vi "Excel - Close Docuement Tests.vi"(8 "error in (no error)":errorcluster) -> (0 "error out":errorcluster)   [LabVIEW 2017]
uses:
  src/LabVIEW NPOI/MS-Excel/MS-Excel.lvclass
  src/LabVIEW NPOI/Document/Document.lvclass
  <vilib>/addons/_JKI Toolkits/Caraya/classes/Test/Test.lvclass
  <vilib>/addons/_JKI Toolkits/Caraya/classes/Assert/Assert.lvclass
  <vilib>/addons/_JKI Toolkits/Caraya/classes/Assert/Assert Not Error.vi
  <vilib>/addons/_JKI Toolkits/Caraya/classes/Assert/Assert True.vi
  D:/Benjamin/Documents/Perso/Code/WC/LabVIEW_NPOI/src/LabVIEW NPOI/Document/Document.lvclass
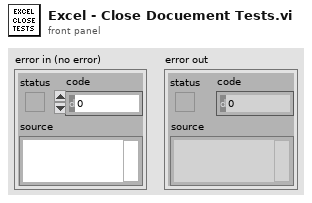
[diagram p1: front panel]
types:
  T1 = enum16{"open", "replace", "create", "open or create", "replace or create", "replace or create with confirmation"}
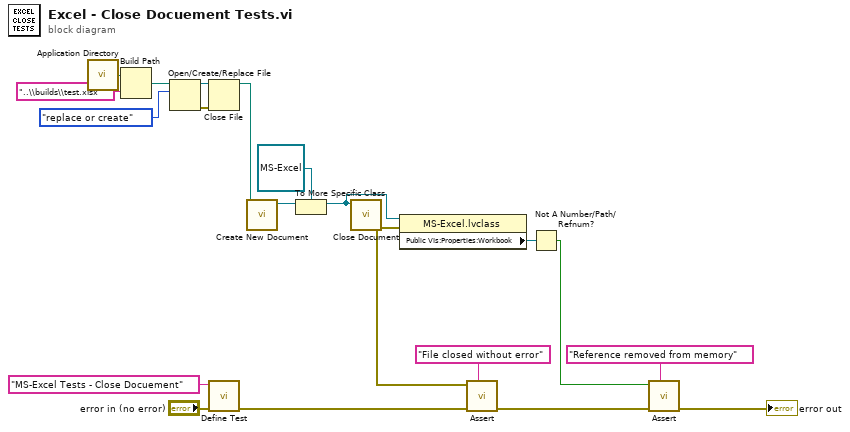
[diagram p0: block diagram]
diagram:
  n1 = call <vilib>:"Application Directory.vi"() -> ("Application Directory"=w6:path)
  n2 = Build Path(base path=w6, name or relative path="..\\builds\\test.xlsx" ("string")) -> (appended path=w4:path)
  n3 = Open/Create/Replace File(file path (use dialog)=w4, operation (0:open)=T1."replace or create") -> (refnum out=w19:refnum<file>, error out=w20:errorcluster)  [unwired: 4 in, 1 out]
  n4 = Close File(refnum=w19, error in=w20) -> (path=w3:path)  [unwired: 1 out]
  n5 = call <vilib>:"Define Test.vi"("error in (no error)"="error in (no error)", "Label (VI Title)"="MS-Excel Tests - Close Docuement") -> ("error out"=w16:errorcluster)  [unwired: 9 in]
  n6 = call "Create New Document.vi"("File Path"=w3) -> ("Document out"=w9:refnum<class "Document.lvclass">)  [unwired: 9 in, 1 out]
  n7 = To More Specific Class(target class=refnum<class "MS-Excel.lvclass"> refnum ("LabVIEW NPOI.lvlib:MS-Excel.lvclass"), reference=w9) -> (specific class reference=w2:refnum<class "MS-Excel.lvclass">)  [unwired: 1 in, 1 out]
  n8 = call "Close Document.vi"("Document in"=w2) -> ("error out"=w10:errorcluster)  [unwired: 10 in]
  n9 = property class="MS-Excel.lvclass"(reference=w2, error in=w10) -> ("Public VIs:Properties:Workbook"=w17:refnum<k24>)  [unwired: 2 out]
  n10 = call-poly <vilib>:"Assert.vi"("Label"="File closed without error", "error in (no error)"=w16, "Not Error?"=w10) -> ("error out"=w13:errorcluster)  [unwired: 8 in]
  n11 = Not A Number/Path/Refnum?(number/path/refnum=w17) -> (NaN/Path/Refnum?=w14:bool)
  n12 = call-poly <vilib>:"Assert.vi"("Label"="Reference removed from memory", "error in (no error)"=w13, "True?"=w14) -> ("error out"=→"error out":errorcluster)  [unwired: 8 in]
